vi "FillianVIconcaten.vi"() -> ()   [LabVIEW 2015]
uses:
  <vilib>/Analysis/Matrix/Datatypes/RealMatrix.ctl
  <vilib>/Utility/error.llb/Error Cluster From Error Code.vi
  <vilib>/ErrorRing/Error Ring.xnode
  <vilib>/Analysis/Matrix/NI_Matrix.lvlib
panel:
  out "appended array":T1
  out "Voltages":sgl[](array[numeric])
  out "Temperatures":dbl[](array[numeric])
  out "Minimum voltage":dbl
  out "Max voltage":dbl
  out "Maximum temp":dbl
  out "Minimum temp":dbl
  out "Mean Temperature":dbl
  out "Mean voltage":dbl
  out "Warnings":errorcluster
  out "temp bat timeout":bool
  out "volt bat timeout":bool
  out "volt link timeout":bool
  out "temp link timeout":bool
  out "Link Quality 2":sgl
  out "Battery Voltage 2":sgl
  out "Battery Voltage":sgl
  out "Link Quality":sgl
  out "Voltage":sgl(graph)
  in  "stop":bool
  out "Temperature":sgl(graph)
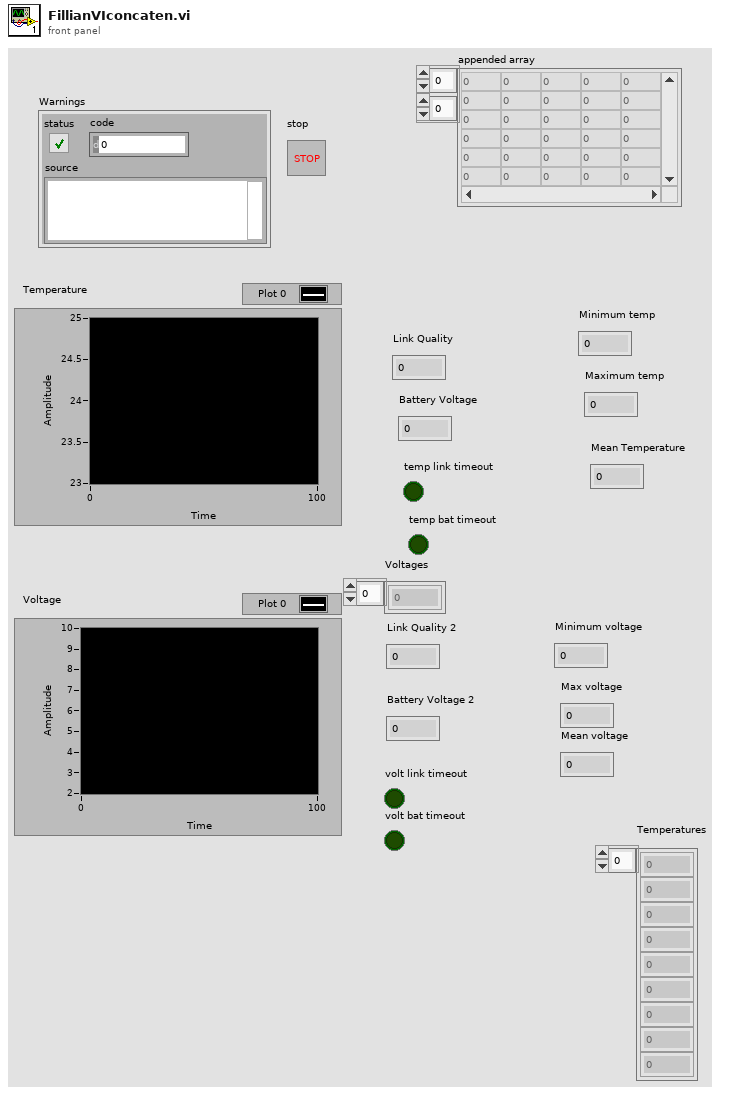
[diagram p1: front panel]
types:
  T1 = typedef "NI_Matrix.lvlib/RealMatrix.ctl" = dbl[][]
  T2 = enum16{"open", "replace", "create", "open or create", "replace or create", "replace or create with confirmation"}
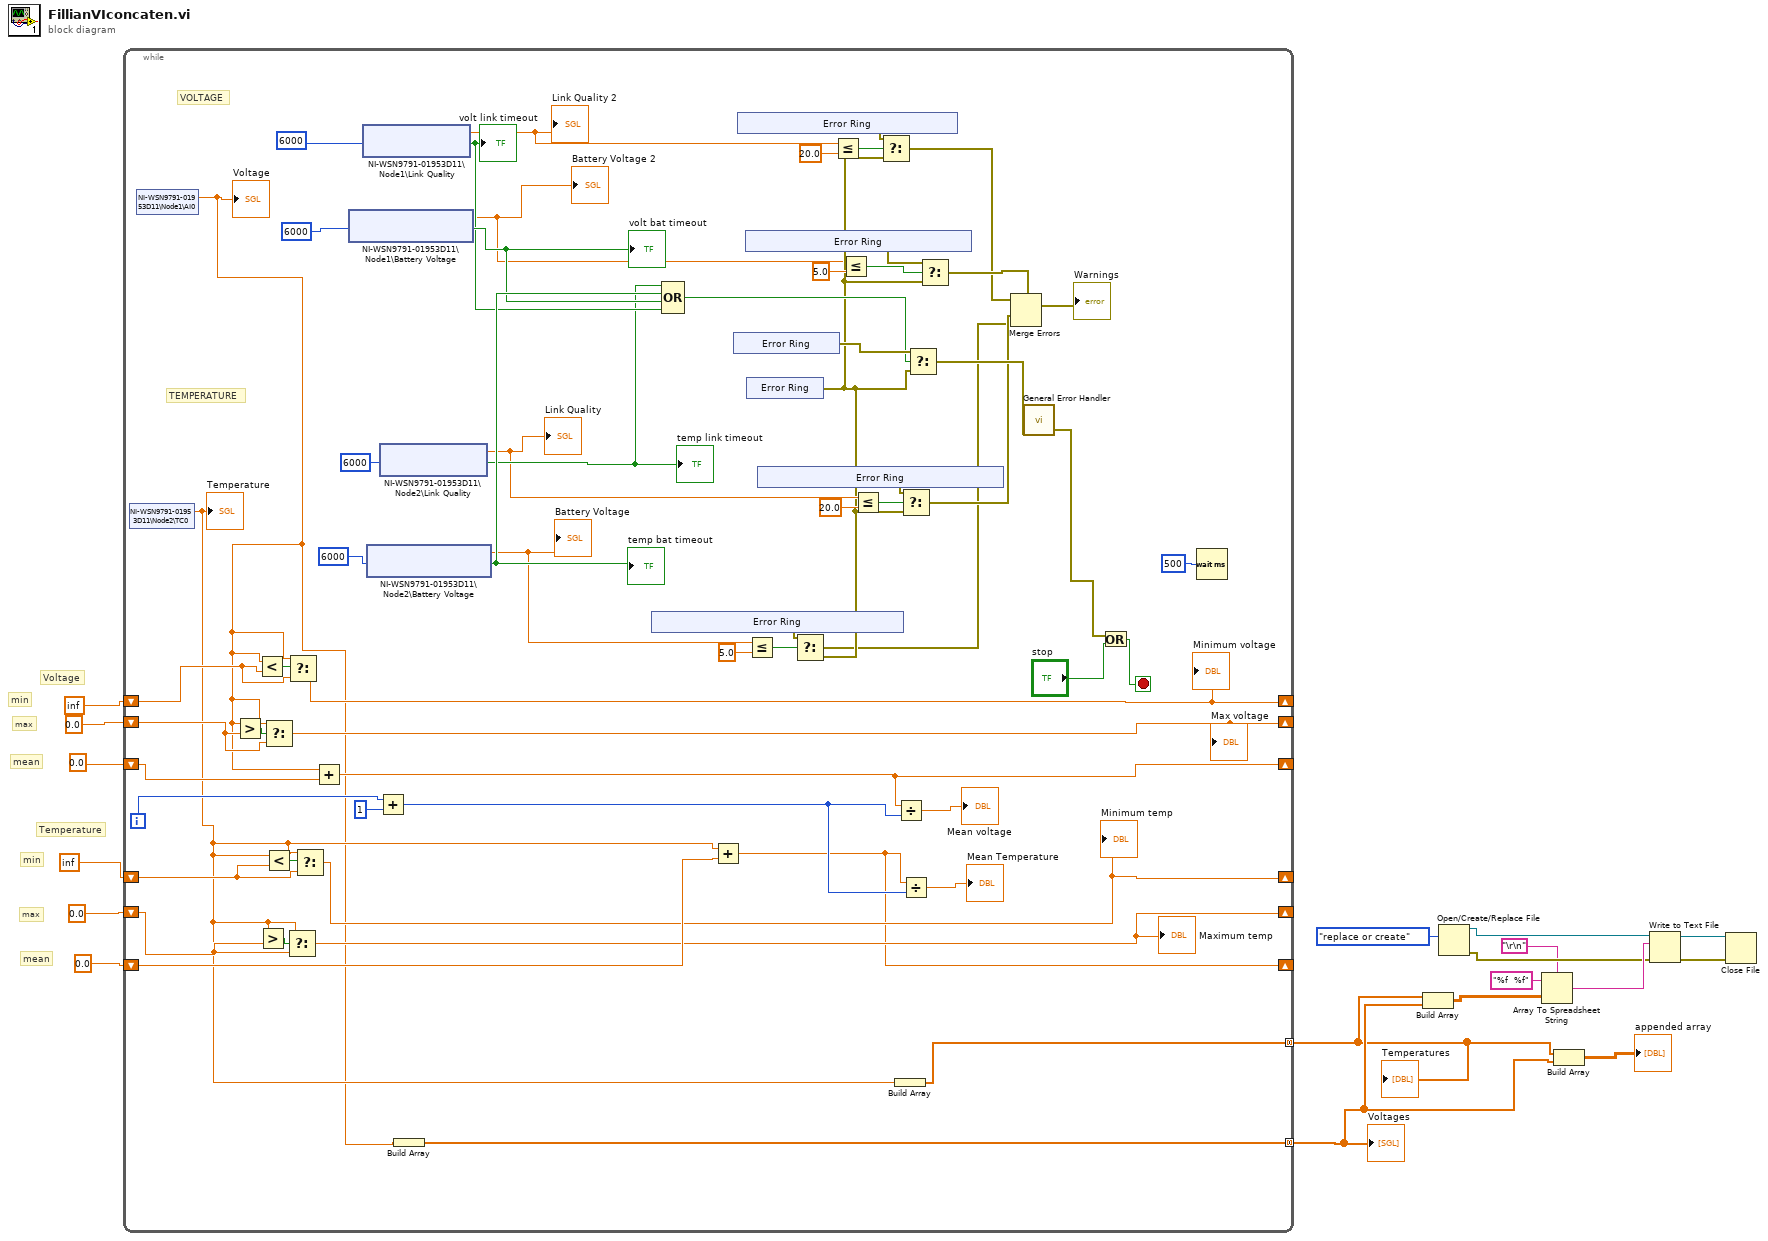
[diagram p0: block diagram]
diagram:
  # "max"
  # "mean"
  # "min"
  # "max"
  # "mean"
  # "min"
  # "Voltage"
  # "Temperature"
  n1 = while {
    shift-right: [w40] -> _
    shift-left: inf -> [w41]
    shift-right: [w43] -> _
    shift-left: 0.0 -> [w38]
    shift-right: [w24] -> _
    shift-left: inf -> [w28]
    shift-right: [w26] -> _
    shift-left: 0.0 -> [w27]
    shift-right: [w36] -> _
    shift-left: 0.0 -> [w39]
    shift-right: [w23] -> _
    shift-left: 0.0 -> [w29]
    tunnel: [w21] -> w2 mode=concatenating
    tunnel: [w19] -> w3 mode=concatenating
    i -> [w34]
    stop <- w69 stop-if-true
    # "VOLTAGE"
    # "TEMPERATURE"
    n2 = shared-variable "NI-WSN9791-01953D11\\Node2\\TC0"() -> (w22:sgl)  [unwired: 1 in, 1 out]
    "Temperature" <- w22
    n3 = shared-variable "NI-WSN9791-01953D11\\Node1\\AI0"() -> (w20:sgl)  [unwired: 1 in, 1 out]
    "Voltage" <- w20
    n4 = Greater?(x=w20, y=w38) -> (0:w44:bool)
    n5 = Less?(x=w20, y=w41) -> (x < y?=w42:bool)
    n6 = Greater?(x=w22, y=w27) -> (0:w31:bool)
    n7 = Select(t=w20, s=w44, f=w38) -> (s? t:f=w43:dbl)
    "Max voltage" <- w43
    n8 = Less?(x=w22, y=w28) -> (x < y?=w32:bool)
    n9 = Select(t=w22, s=w31, f=w27) -> (s? t:f=w26:dbl)
    "Maximum temp" <- w26
    n10 = Select(t=w20, s=w42, f=w41) -> (s? t:f=w40:dbl)
    "Minimum voltage" <- w40
    n11 = Select(t=w22, s=w32, f=w28) -> (s? t:f=w24:dbl)
    "Minimum temp" <- w24
    n12 = Add(x=w20, y=w39) -> (x+y=w36:dbl)
    n13 = shared-variable "NI-WSN9791-01953D11\\Node1\\Battery Voltage"(6000 ("ms timeout (0)")) -> (w37:sgl, w74:bool)  [unwired: 1 in, 1 out]
    "Battery Voltage 2" <- w37
    "volt bat timeout" <- w74
    n14 = shared-variable "NI-WSN9791-01953D11\\Node1\\Link Quality"(6000 ("ms timeout (0)")) -> (w58:sgl, w73:bool)  [unwired: 1 in, 1 out]
    "Link Quality 2" <- w58
    "volt link timeout" <- w73
    n15 = shared-variable "NI-WSN9791-01953D11\\Node2\\Battery Voltage"(6000 ("ms timeout (0)")) -> (w47:sgl, w75:bool)  [unwired: 1 in, 1 out]
    "Battery Voltage" <- w47
    "temp bat timeout" <- w75
    n16 = Add(x=w34, y=1) -> (x+y=w30:i32)
    n17 = shared-variable "NI-WSN9791-01953D11\\Node2\\Link Quality"(6000 ("ms timeout (0)")) -> (w65:sgl, w66:bool)  [unwired: 1 in, 1 out]
    "Link Quality" <- w65
    "temp link timeout" <- w66
    n18 = Build Array(w20) -> (w19:sgl[])
    n19 = xnode "Error Ring"() -> ("error out"=w48:errorcluster)
    n20 = Compound Arithmetic op=OR(w66, w75, w74, w73) -> (w70:bool)
    n21 = Add(x=w22, y=w29) -> (x+y=w23:dbl)
    n22 = xnode "Error Ring"() -> ("error out"=w72:errorcluster)
    n23 = xnode "Error Ring"() -> ("error out"=w59:errorcluster)
    n24 = xnode "Error Ring"() -> ("error out"=w55:errorcluster)
    n25 = xnode "Error Ring"() -> ("error out"=w46:errorcluster)
    n26 = Less Or Equal?(x=w47, y=sgl 5.0) -> (x <= y?=w49:bool)
    n27 = xnode "Error Ring"() -> ("error out"=w62:errorcluster)
    n28 = Select(t=w48, s=w49, f=w46) -> (s? t:f=w45:errorcluster)
    n29 = Less Or Equal?(x=w58, y=sgl 20.0) -> (x <= y?=w60:bool)
    n30 = Less Or Equal?(x=w37, y=sgl 5.0) -> (x <= y?=w56:bool)
    n31 = Less Or Equal?(x=w65, y=sgl 20.0) -> (x <= y?=w63:bool)
    n32 = Select(t=w59, s=w60, f=w46) -> (s? t:f=w53:errorcluster)
    n33 = Build Array(w22) -> (w21:sgl[])
    n34 = Divide(x=w36, y=w30) -> (x/y=→"Mean voltage":dbl)
    n35 = Select(t=w62, s=w63, f=w46) -> (s? t:f=w51:errorcluster)
    n36 = Divide(x=w23, y=w30) -> (x/y=→"Mean Temperature":dbl)
    n37 = Select(t=w72, s=w70, f=w46) -> (s? t:f=w71:errorcluster)
    n38 = Select(t=w55, s=w56, f=w46) -> (s? t:f=w54:errorcluster)
    n39 = Merge Errors(w53, w54, w51, w45) -> (→"Warnings":errorcluster)
    n40 = call <vilib>:"General Error Handler.vi"("error in (no error)"=w71) -> ("error out"=w67:errorcluster)  [unwired: 10 in, 4 out]
    n41 = Or(x=w67, y="stop") -> (x .or. y?=w69:bool)
    n42 = Wait (ms)(milliseconds to wait=u32 500) -> ()  [unwired: 1 out]
  }
  "Temperatures" <- w2
  "Voltages" <- w3
  n43 = Build Array(w2, w3) -> (w1:sgl[][])
  n44 = Open/Create/Replace File(operation (0:open)=T2."replace or create") -> (refnum out=w10:refnum<file>, error out=w9:errorcluster)  [unwired: 5 in, 1 out]
  n45 = Array To Spreadsheet String(delimiter (Tab)="\r\n", array=w1, 3:"%f  %f" ("format string")) -> (spreadsheet string=w11:string)
  n46 = Build Array(w2, w3) -> (→"appended array":T1)
  n47 = Write to Text File(file (use dialog)=w10, text=w11, error in=w9) -> (refnum out=w8:refnum<file>, error out=w7:errorcluster)  [unwired: 1 in, 1 out]
  n48 = Close File(refnum=w8, error in=w7) -> ()  [unwired: 2 out]
